vi "low_rate_processing.vi"(0 "Reset":bool, 2 "Config":T1={"I/O"={"Buffering (in/out)"=[1.9, 6.0], "Output Device"=1, "Sound"={"sample rate (S/s)"=96000.0, "number of channels"=2, "bits per sample"=24}, "Input Device"=4}, "Noise limit low"=101.5, "Distortion LF cut"=101.5, "Averaging Tc"=3.0, "High rate STFT"={"Win param"=101.5, "Window type"=61, "Win order"=2, "DFT size"=64, "Channels"=[7], "Oversample"=64}, "Low rate STFT"={"Win param"=120.0, "Window type"=61, "Win order"=8, "DFT size"=64, "Channels"=[7], "Oversample"=64}, "Hum filter"={"Frequency"=0.0, "Tc"=0.0}, "KF params"={"Process n"=101.5}} {"Low rate STFT"."Oversample" min=1 step=1; "Low rate STFT"."Channels" min=0 step=1; "Low rate STFT"."DFT size" min=1 step=1; "Low rate STFT"."Window type" items=["Rectangle"=0, "Hanning"=1, "Hamming"=2, "Blackman-Harris"=3, "Exact Blackman"=4, "Blackman"=5, "Flat Top"=6, "4 Term B-Harris "=7, "7 Term B-Harris"=8, "Low Sidelobe"=9, "Blackman Nuttall"=11, "Triangle"=30, "Bartlett-Hanning"=31, "Bohman"=32, "Parzen"=33, "Welch"=34, "Kaiser"=60, "Dolph-Chebyshev"=61, "Gaussian"=62]; "High rate STFT"."Oversample" min=1 step=1; "High rate STFT"."Channels" min=0 step=1; "High rate STFT"."DFT size" min=1 step=1; "High rate STFT"."Window type" items=["Rectangle"=0, "Hanning"=1, "Hamming"=2, "Blackman-Harris"=3, "Exact Blackman"=4, "Blackman"=5, "Flat Top"=6, "4 Term B-Harris "=7, "7 Term B-Harris"=8, "Low Sidelobe"=9, "Blackman Nuttall"=11, "Triangle"=30, "Bartlett-Hanning"=31, "Bohman"=32, "Parzen"=33, "Welch"=34, "Kaiser"=60, "Dolph-Chebyshev"=61, "Gaussian"=62]; "I/O"."Input Device" format="%.0x"; "I/O"."Output Device" format="%.0x"}, 4 "Modulation info":T5={"Fs full"=0.0, "Fs high"=0.0, "Fs low"=0.0, "Read size"=0, "FFT size low"=5000, "df low"=5000.0, "High carriers"=[], "Low carriers"=[], "Hi channels at low"=[7]} {"Hi channels at low" min=0 step=1; "Low carriers" format="%#_6p"; "High carriers" format="%#_6p"}, 11 "Raw data":dbl[][](array[numeric])) -> (26 "Prev carrier amplitude":cdb[][](array[numeric]) format="%#_3p")   [LabVIEW 2014]
uses:
  modulation_info.ctl
  ilemt_config.ctl
  <vilib>/sound2/lvsound2.llb/Sound Data Format.ctl
  stft_params.ctl
  <vilib>/Analysis/4window.llb/windowTd.ctl
  <vilib>/Analysis/NI_AALPro.lvlib
panel:
  # "High"
  # "Low"
  # "Signal/reference"
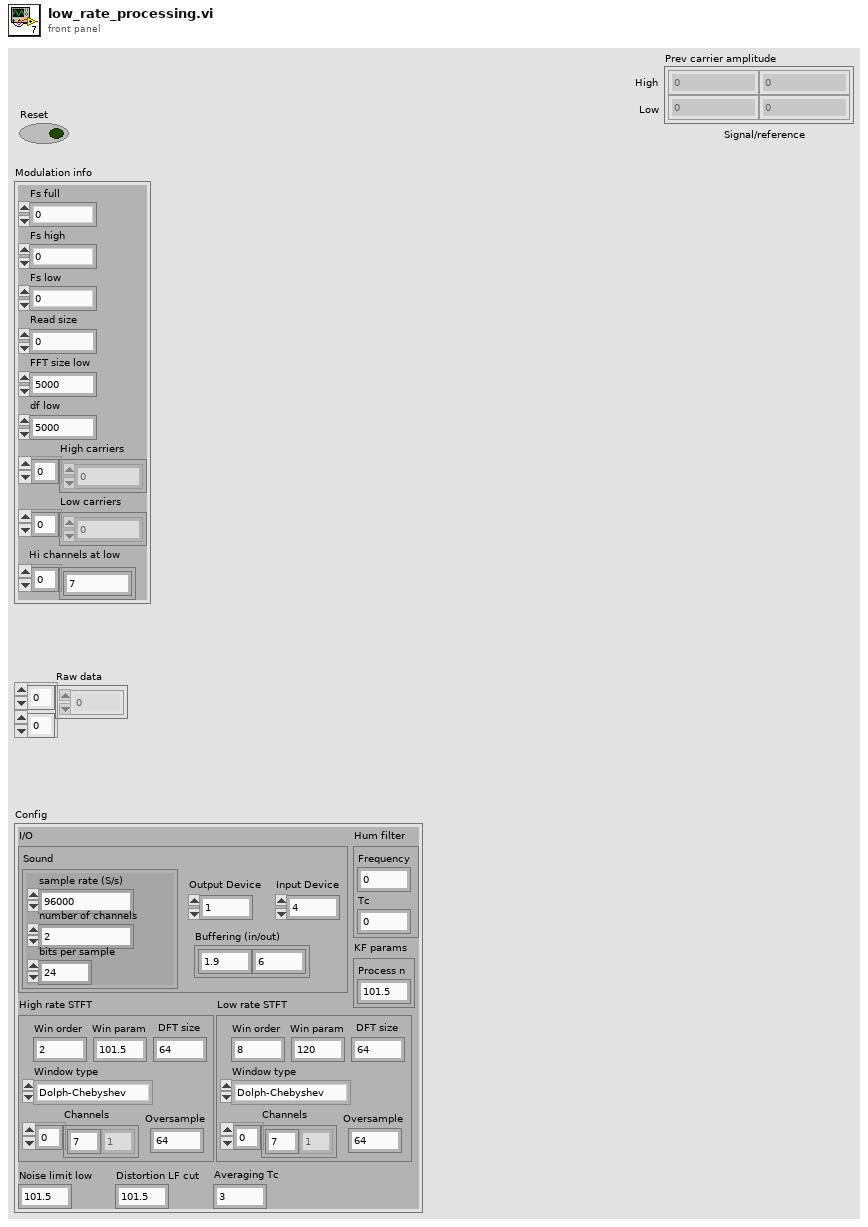
[diagram p1: front panel]
types:
  T1 = typedef "ilemt_config.ctl" = cluster{"I/O":cluster{"Buffering (in/out)":dbl[], "Output Device":u32, "Sound":T2, "Input Device":u32}, "Noise limit low":dbl, "Distortion LF cut":dbl, "Averaging Tc":sgl, "High rate STFT":T3, "Low rate STFT":T3, "Hum filter":cluster{"Frequency":dbl, "Tc":dbl}, "KF params":cluster{"Process n":dbl}}
  T2 = typedef "Sound Data Format.ctl" = cluster{"sample rate (S/s)":dbl, "number of channels":i32, "bits per sample":i32}
  T3 = typedef "stft_params.ctl" = cluster{"Win param":dbl, "Window type":T4, "Win order":i32, "DFT size":i32, "Channels":i32[], "Oversample":i32}
  T4 = typedef "NI_AALPro.lvlib/windowTd.ctl" = u32
  T5 = typedef "modulation_info.ctl" = cluster{"Fs full":dbl, "Fs high":dbl, "Fs low":dbl, "Read size":i32, "FFT size low":i32, "df low":dbl, "High carriers":dbl[], "Low carriers":dbl[], "Hi channels at low":i32[]}
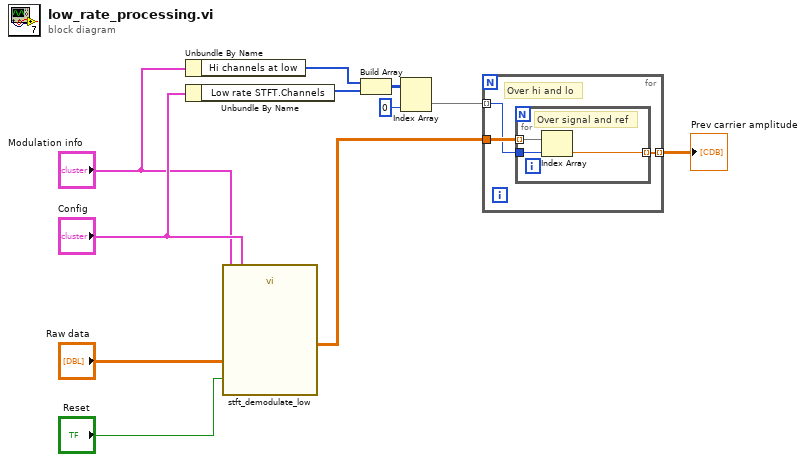
[diagram p0: block diagram]
diagram:
  n1 = Unbundle By Name("Modulation info") -> ("Hi channels at low"=w7:i32[])
  n2 = Unbundle By Name("Config") -> ("Low rate STFT.Channels"=w10:i32[])
  n3 = call "stft_demodulate_low.vi"("Reset"="Reset", "Config"="Config", "Modulation info"="Modulation info", "Raw data"="Raw data") -> ("STFT"=w2:cdb[][])  [unwired: 6 in, 1 out]
  n4 = Build Array(w7, w10) -> (w9:i32[][])
  n5 = Index Array(array=w9, index (col)=0 ("disabled index (col)")) -> (element=w11:i32[])  [unwired: 1 in]
  n6 = for {
    tunnel: w2 -> [w14]
    tunnel: w11 -> [w13] mode=indexing
    tunnel: [w12] -> w6 mode=indexing
    # "Over hi and lo"
    n7 = for {
      tunnel: w14 -> [w17] mode=indexing
      tunnel: w13 -> [w16]
      tunnel: [w15] -> w12 mode=indexing
      # "Over signal and ref"
      n8 = Index Array(array=w17, index=w16) -> (element=w15:cdb)
    }
  }
  "Prev carrier amplitude" <- w6
